vi "Get Piece Coordinates.vi"(8 "error in (no error)":errorcluster, 11 "object in":refnum<class "Piece of Bricks.lvclass">) -> (0 "error out":errorcluster, 2 "Piece Coordinates":T1[](array[typedef]), 3 "object out":refnum<class "Piece of Bricks.lvclass">)   [LabVIEW 2017, in "Piece of Bricks.lvclass"]
uses:
  Piece of Bricks.lvclass
  Controls/Coordinates.ctl
  Piece of Bricks.lvclass/Piece of Bricks.ctl
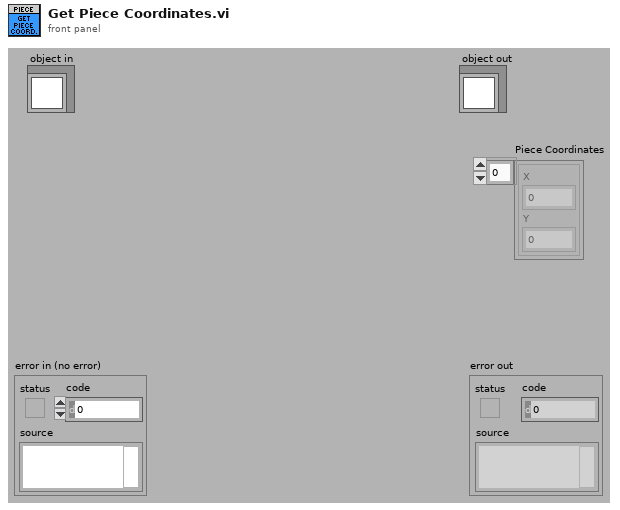
[diagram p1: front panel]
types:
  T1 = typedef "Coordinates.ctl" = cluster{"X":i32, "Y":i32}
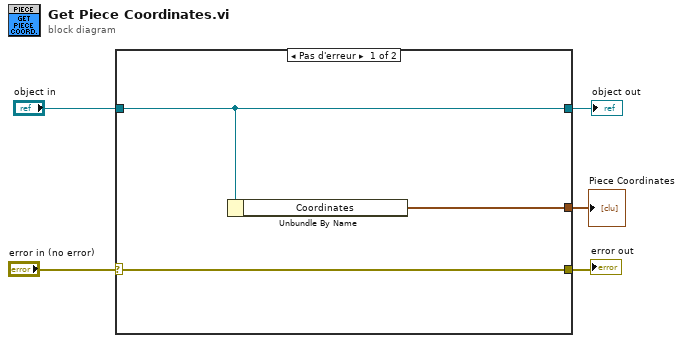
[diagram p0: block diagram]
diagram:
  n1 = case shown="Pas d'erreur" "error in (no error)" {
    selector: "error in (no error)" -> [w7 w10]
    tunnel: [w7 w10] -> w4
    tunnel: [w6 w9] -> w2
    tunnel: "object in" -> [w6 w9]
    tunnel: [w8 _] -> w1
    frame No Error {
      n2 = Unbundle By Name(w6) -> ("Coordinates"=w8:T1[])
    }
    frame Error {
    }
  }
  "error out" <- w4
  "object out" <- w2
  "Piece Coordinates" <- w1
